vi "dfd_X Equal NaN Inf Zero.vi"(11 "roots":cdb[](array[numeric])) -> (1 "contain zero ?":bool, 2 "contain Inf ?":bool, 3 "contain NaN ?":bool)   [LabVIEW 2017, in "NI_DigFilterLicensed.lvlib"]
uses:
  <vilib>/addons/Digital Filter Design/NI_DigFilterLicensed.lvlib
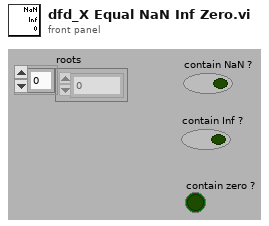
[diagram p1: front panel]
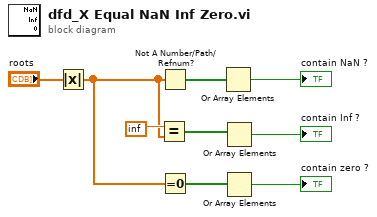
[diagram p0: block diagram]
diagram:
  n1 = Absolute Value(x="roots") -> (abs(x)=w2:dbl[])
  n2 = Equal?(x=inf, y=w2) -> (x = y?=w3:bool[])
  n3 = Not A Number/Path/Refnum?(number/path/refnum=w2) -> (NaN/Path/Refnum?=w5:bool[])
  n4 = Equal To 0?(x=w2) -> (x = 0?=w1:bool[])
  n5 = Or Array Elements(Boolean array=w5) -> (logical OR=→"contain NaN ?":bool)
  n6 = Or Array Elements(Boolean array=w3) -> (logical OR=→"contain Inf ?":bool)
  n7 = Or Array Elements(Boolean array=w1) -> (logical OR=→"contain zero ?":bool)
